vi "FGV.vi"(9 "command":string, 10 "functions":T1(ring), 11 "response to save":string) -> (2 "Variant":variant, 3 "response retrirvrd":string)   [LabVIEW 2019, in "simulado.lvclass"]
uses:
  simulado.lvclass
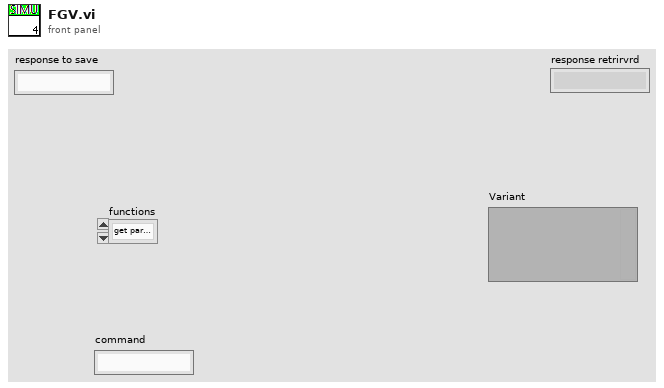
[diagram p1: front panel]
types:
  T1 = enum16{"get parameter", "Set parameters", "reset parameter", ""}
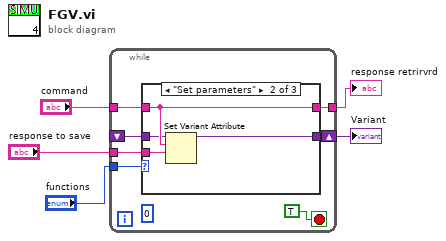
[diagram p0: block diagram]
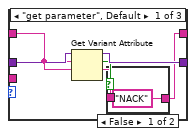
[diagram p2: hidden frame]
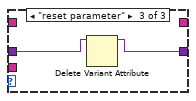
[diagram p4: hidden frame]
diagram:
  n1 = while {
    tunnel: "functions" -> [w12]
    tunnel: "command" -> [w11]
    tunnel: [w10] -> w3
    tunnel: "response to save" -> [w8]
    shift-right: [w7] -> w1
    shift-left: _ -> [w6]
    stop <- TRUE stop-if-true
    (unwired) 0
    n2 = case shown="\"Set parameters\"" w12 {
      tunnel: w11 -> [w16 w23 _]
      tunnel: [w13 w23 _] -> w10
      tunnel: w8 -> [_ w24 _]
      tunnel: [w17 w22 w25] -> w7
      tunnel: w6 -> [w18 w21 w26]
      frame "get parameter", Default {
        n3 = Get Variant Attribute(Variant=w18, name=w16, default value (empty Variant)=w16) -> (duplicate Variant=w17:variant, found=w15:bool, value=w14:string)  [unwired: 1 in, 1 out]
        n4 = case shown="False" w15 {
          tunnel: w14 -> [_ w20]
          tunnel: ["NACK" ("command") w20] -> w13
          frame False {
          }
          frame True {
          }
        }
      }
      frame "Set parameters" {
        n5 = Set Variant Attribute(Variant=w21, name=w23, value=w24) -> (Variant out=w22:variant)  [unwired: 1 in, 2 out]
      }
      frame "reset parameter" {
        n6 = Delete Variant Attribute(7:w26) -> (3:w25:variant)  [unwired: 2 in, 2 out]
      }
    }
  }
  "response retrirvrd" <- w3
  "Variant" <- w1
